vi "Generate Specific Result.vi"(8 "error in (no error)":errorcluster, 10 "Test Method":T4) -> (0 "error out":errorcluster, 3 "Data":T1[](array[typedef])=[{"Name"="Test Case.lvclass:Test Failing Test.vi", "Description"="Description", "Status"=enum."Failed", "Result Type"=enum."Fail", "Execution Time"=0.0, "Data"={"Expected"=variant, "Actual"=variant, "Delta"=variant}}, {"Name"="Test Case.lvclass:Test Failing Test.vi", "Description"="Failed:\nDescription\nMessage", "Status"=enum."Failed", "Result Type"=enum."Test Case", "Execution Time"=0.013, "Data"={"Expected"=variant, "Actual"=variant, "Delta"=variant}}, {"Name"="Test Case.lvclass:Test Passing Test.vi", "Description"="Description", "Status"=enum."Passed", "Result Type"=enum."Pass", "Execution Time"=0.0, "Data"={"Expected"=variant, "Actual"=variant, "Delta"=variant}}, {"Name"="Test Case.lvclass:Test Passing Test.vi", "Description"="Passed:\nDescription\nMessage", "Status"=enum."Passed", "Result Type"=enum."Test Case", "Execution Time"=0.022, "Data"={"Expected"=variant, "Actual"=variant, "Delta"=variant}}, {"Name"="Test Case.lvclass", "Description"="", "Status"=enum."Failed", "Result Type"=enum."Test Suite", "Execution Time"=0.0, "Data"={"Expected"=variant, "Actual"=variant, "Delta"=variant}}, {"Name"="Test Suite", "Description"="", "Status"=enum."Failed", "Result Type"=enum."Test Suite", "Execution Time"=0.0, "Data"={"Expected"=variant, "Actual"=variant, "Delta"=variant}}])   [LabVIEW 2020, in "Text Report Test.lvclass"]
uses:
  Text Report Test.lvclass
  source/Core/Result/Result.ctl
  source/Core/Result/Status.ctl
  source/Core/Result/Type.ctl
  Test Doubles/Test Case Test Double/Methods.ctl
  Test Doubles/Test Case Test Double/Test Case Test Double.lvclass
  source/Core/Result/Result.lvlib
  source/LUnit Test Case.lvclass
panel:
  out "Results":cluster{"Results":T1[]}[](array[cluster])
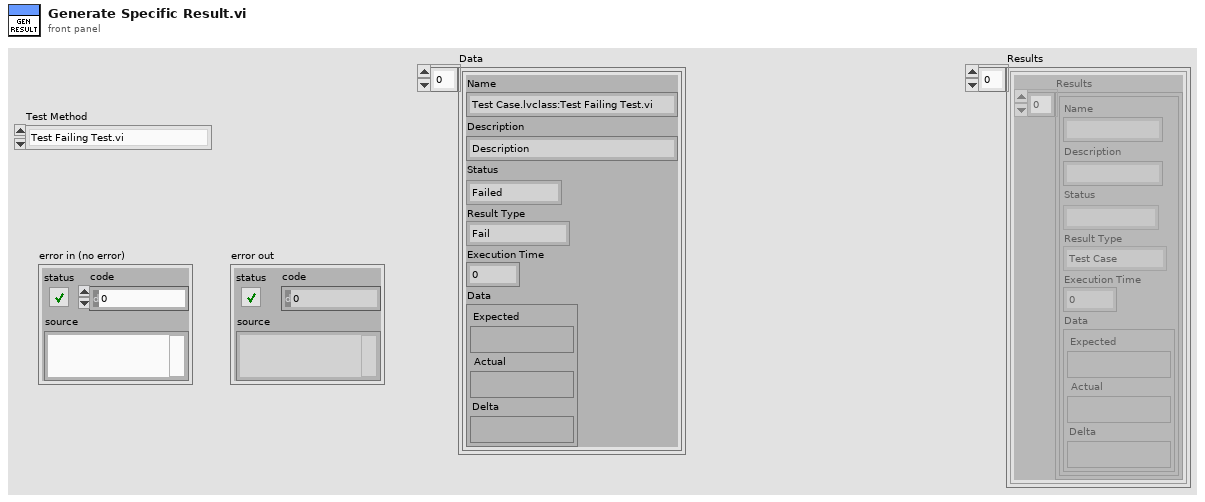
[diagram p1: front panel]
types:
  T1 = typedef "Result.lvlib/Result.ctl" = cluster{"Name":string, "Description":string, "Status":T2, "Result Type":T3, "Execution Time":dbl, "Data":cluster{"Expected":variant, "Actual":variant, "Delta":variant}}
  T2 = typedef "Result.lvlib/Status.ctl" = enum16{"", "Passed", "Failed", "Error", "Skipped", "Setup Error", "Broken", "Teardown Error"}
  T3 = typedef "Result.lvlib/Type.ctl" = enum16{"Test Case", "Test Suite", "Test Run", "Pass", "Fail", "Skip", "Pass if", "Fail if", "Pass if Error", "Fail if Error", "Pass if Equal", "Fail if Equal"}
  T4 = typedef "Test Case Test Double.lvclass/Methods.ctl" = enum16{"Test Failing Test.vi", "Test Passing Test.vi", "Test Error Test.vi", "Test Skip Test.vi", "Test Passing Pass If Test.vi", "Test Failing Pass If Test.vi", "Test Failing Fail If Test.vi", "Test Passing Fail If Test.vi", "Test Passing Pass If Error Test.vi", "Test Failing Pass If Error Test.vi", "Test Passing Fail If Error Test.vi", "Test Failing Fail If Error Test.vi", "Test Passing Pass If Equal Test.vi", "Test Failing Pass If Equal Test.vi", "Test Failing Fail If Equal Test.vi", "Test Passing Fail If Equal Test.vi", "Freezing Test.vi", "Test Pass on Expected Error Code.vi", "Test Error on Unexpected Error Code.vi", "Test Fail on Expected Error Code.vi", "Test Error when Fail on Unexpected Error Code.vi", "Test Pass on Expected Element in Array.vi", "Test Fail on Expected Element Not in Array.vi", "Test Pass on Expected Element in Set.vi", "Test Fail on Expected Element Not in Set.vi", "Test Pass on Expected Element in Map.vi", "Test Fail on Expected Element Not in Map.vi", "Test Fail on Unexpected Element in Array.vi", "Test Pass on Unexpected Element Not in Array.vi", "Test Fail if Unexpected Element in Set.vi", "Test Pass if Unexpected Element Not in Set.vi", "Test Fail if Unexpected Element in Map.vi", "Test Pass if Unexpected Element Not in Map.vi", "Test Pass on Expected Element in Array of Clusters.vi", "Test Pass on Expected Element Not in Array of Clusters.vi", "Test Matching String Test.vi", "Test Not Matching String Test.vi", "Verify Passing.vi", "Without Prefix.vi", "Private VI.vi"}
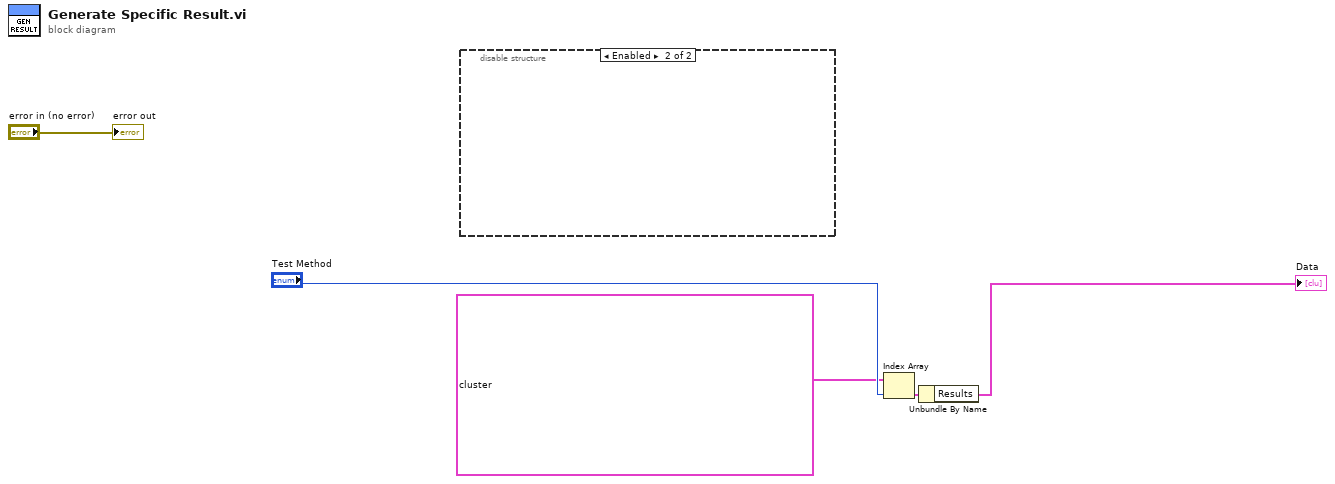
[diagram p0: block diagram]
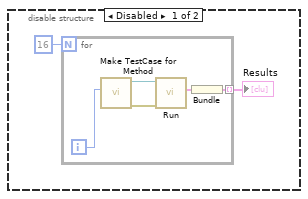
[diagram p2: hidden frame]
diagram:
  n1 = disable-structure shown="Enabled" {
    frame Disabled {
      n2 = for {
        N: 16 -> [_]
        tunnel: [w9] -> w6 mode=indexing
        i -> [w10]
        n3 = call "Make TestCase for Method.vi"("Test Method"=w10) -> ("error out"=w11:errorcluster, "LUnit Test Case V2 out"=w12:refnum<class "LUnit Test Case.lvclass">)  [unwired: 9 in]
        n4 = call-dynamic "Run.vi"("error in (no error)"=w11, "LUnit Test Case In"=w12) -> ("Results"=w8:T1[])  [unwired: 6 in, 3 out]
        n5 = Bundle("Results"=w8) -> (w9:cluster{"Results":T1[]})  [unwired: 1 in]
      }
      "Results" <- w6
    }
    frame Enabled {
    }
  }
  n6 = Index Array(array=cluster{"Results":T1[]}[] [{"Results"=[{"Name"="Test Case Test Double.lvclass:Test Failing Test.vi", "Description"="Description", "Status"=enum."Failed", "Result Type"=enum."Fail", "Execution Time"=0.0, "Data"={"Expected"=variant, "Actual"=variant, "Delta"=variant}}, {"Name"="Test Case Test Double.lvclass:Test Failing Test.vi", "Description"="Failed:\nMessage", "Status"=enum."Failed", "Result Type"=enum."Test Case", "Execution Time"=0.067, "Data"={"Expected"=variant, "Actual"=variant, "Delta"=variant}}]}, {"Results"=[{"Name"="Test Case Test Double.lvclass:Test Passing Test.vi", "Description"="", "Status"=enum."Passed", "Result Type"=enum."Pass", "Execution Time"=0.0, "Data"={"Expected"=variant, "Actual"=variant, "Delta"=variant}}, {"Name"="Test Case Test Double.lvclass:Test Passing Test.vi", "Description"="Passed", "Status"=enum."Passed", "Result Type"=enum."Test Case", "Execution Time"=0.051, "Data"={"Expected"=variant, "Actual"=variant, "Delta"=variant}}]}, {"Results"=[{"Name"="Test Case Test Double.lvclass:Test Error Test.vi", "Description"="Source", "Status"=enum."Error", "Result Type"=enum."Test Case", "Execution Time"=0.0, "Data"={"Expected"=variant, "Actual"=variant, "Delta"=variant}}]}, {"Results"=[{"Name"="Test Case Test Double.lvclass:Test Skip Test.vi", "Description"="Description", "Status"=enum."Skipped", "Result Type"=enum."Skip", "Execution Time"=0.0, "Data"={"Expected"=variant, "Actual"=variant, "Delta"=variant}}, {"Name"="Test Case Test Double.lvclass:Test Skip Test.vi", "Description"="Skipped:\nDescription\nMessage", "Status"=enum."Skipped", "Result Type"=enum."Test Case", "Execution Time"=0.07, "Data"={"Expected"=variant, "Actual"=variant, "Delta"=variant}}]}, {"Results"=[{"Name"="Test Case Test Double.lvclass:Test Passing Pass If Test.vi", "Description"="Description", "Status"=enum."Passed", "Result Type"=enum."Pass if", "Execution Time"=0.0, "Data"={"Expected"=variant, "Actual"=variant, "Delta"=variant}}, {"Name"="Test Case Test Double.lvclass:Test Passing Pass If Test.vi", "Description"="Passed:\nDescription\nMessage", "Status"=enum."Passed", "Result Type"=enum."Test Case", "Execution Time"=0.048, "Data"={"Expected"=variant, "Actual"=variant, "Delta"=variant}}]}, {"Results"=[{"Name"="Test Case Test Double.lvclass:Test Failing Pass If Test.vi", "Description"="Description", "Status"=enum."Failed", "Result Type"=enum."Pass if", "Execution Time"=0.0, "Data"={"Expected"=variant, "Actual"=variant, "Delta"=variant}}, {"Name"="Test Case Test Double.lvclass:Test Failing Pass If Test.vi", "Description"="Failed:\nDescription\nMessage", "Status"=enum."Failed", "Result Type"=enum."Test Case", "Execution Time"=0.042, "Data"={"Expected"=variant, "Actual"=variant, "Delta"=variant}}]}, {"Results"=[{"Name"="Test Case Test Double.lvclass:Test Failing Fail If Test.vi", "Description"="Description", "Status"=enum."Failed", "Result Type"=enum."Fail if", "Execution Time"=0.0, "Data"={"Expected"=variant, "Actual"=variant, "Delta"=variant}}, {"Name"="Test Case Test Double.lvclass:Test Failing Fail If Test.vi", "Description"="Failed:\nDescription\nMessage", "Status"=enum."Failed", "Result Type"=enum."Test Case", "Execution Time"=0.05, "Data"={"Expected"=variant, "Actual"=variant, "Delta"=variant}}]}, {"Results"=[{"Name"="Test Case Test Double.lvclass:Test Passing Fail If Test.vi", "Description"="Description", "Status"=enum."Passed", "Result Type"=enum."Fail if", "Execution Time"=0.0, "Data"={"Expected"=variant, "Actual"=variant, "Delta"=variant}}, {"Name"="Test Case Test Double.lvclass:Test Passing Fail If Test.vi", "Description"="Passed:\nDescription\nMessage", "Status"=enum."Passed", "Result Type"=enum."Test Case", "Execution Time"=0.052, "Data"={"Expected"=variant, "Actual"=variant, "Delta"=variant}}]}, {"Results"=[{"Name"="Test Case Test Double.lvclass:Test Passing Pass If Error Test.vi", "Description"="Description", "Status"=enum."Passed", "Result Type"=enum."Pass if Error", "Execution Time"=0.0, "Data"={"Expected"=variant, "Actual"=variant, "Delta"=variant}}, {"Name"="Test Case Test Double.lvclass:Test Passing Pass If Error Test.vi", "Description"="Passed:\nDescription\nError 42 occured: \"Error\"", "Status"=enum."Passed", "Result Type"=enum."Test Case", "Execution Time"=0.037, "Data"={"Expected"=variant, "Actual"=variant, "Delta"=variant}}]}, {"Results"=[{"Name"="Test Case Test Double.lvclass:Test Failing Pass If Error Test.vi", "Description"="Description", "Status"=enum."Failed", "Result Type"=enum."Pass if Error", "Execution Time"=0.0, "Data"={"Expected"=variant, "Actual"=variant, "Delta"=variant}}, {"Name"="Test Case Test Double.lvclass:Test Failing Pass If Error Test.vi", "Description"="Failed:\nDescription\nNo error occured.", "Status"=enum."Failed", "Result Type"=enum."Test Case", "Execution Time"=0.043, "Data"={"Expected"=variant, "Actual"=variant, "Delta"=variant}}]}, {"Results"=[{"Name"="Test Case Test Double.lvclass:Test Passing Fail If Error Test.vi", "Description"="Description", "Status"=enum."Passed", "Result Type"=enum."Fail if Error", "Execution Time"=0.0, "Data"={"Expected"=variant, "Actual"=variant, "Delta"=variant}}, {"Name"="Test Case Test Double.lvclass:Test Passing Fail If Error Test.vi", "Description"="Passed:\nDescription\nNo error occured.", "Status"=enum."Passed", "Result Type"=enum."Test Case", "Execution Time"=0.042, "Data"={"Expected"=variant, "Actual"=variant, "Delta"=variant}}]}, {"Results"=[{"Name"="Test Case Test Double.lvclass:Test Failing Fail If Error Test.vi", "Description"="Description", "Status"=enum."Failed", "Result Type"=enum."Fail if Error", "Execution Time"=0.0, "Data"={"Expected"=variant, "Actual"=variant, "Delta"=variant}}, {"Name"="Test Case Test Double.lvclass:Test Failing Fail If Error Test.vi", "Description"="Failed:\nDescription\nError 42 occured: \"Error\"", "Status"=enum."Failed", "Result Type"=enum."Test Case", "Execution Time"=0.036, "Data"={"Expected"=variant, "Actual"=variant, "Delta"=variant}}]}, {"Results"=[{"Name"="Test Case Test Double.lvclass:Test Passing Pass If Equal Test.vi", "Description"="Description", "Status"=enum."Passed", "Result Type"=enum."Pass if Equal", "Execution Time"=0.0, "Data"={"Expected"=variant, "Actual"=variant, "Delta"=variant}}, {"Name"="Test Case Test Double.lvclass:Test Passing Pass If Equal Test.vi", "Description"="Passed:\nDescription\nExpected: Equal\nActual:   Equal", "Status"=enum."Passed", "Result Type"=enum."Test Case", "Execution Time"=0.056, "Data"={"Expected"=variant, "Actual"=variant, "Delta"=variant}}]}, {"Results"=[{"Name"="Test Case Test Double.lvclass:Test Failing Pass If Equal Test.vi", "Description"="Description", "Status"=enum."Failed", "Result Type"=enum."Pass if Equal", "Execution Time"=0.0, "Data"={"Expected"=variant, "Actual"=variant, "Delta"=variant}}, {"Name"="Test Case Test Double.lvclass:Test Failing Pass If Equal Test.vi", "Description"="Failed:\nDescription\nExpected: Equal\nActual:   Not Equal", "Status"=enum."Failed", "Result Type"=enum."Test Case", "Execution Time"=0.045, "Data"={"Expected"=variant, "Actual"=variant, "Delta"=variant}}]}, {"Results"=[{"Name"="Test Case Test Double.lvclass:Test Failing Fail If Equal Test.vi", "Description"="Description", "Status"=enum."Failed", "Result Type"=enum."Fail if Equal", "Execution Time"=0.0, "Data"={"Expected"=variant, "Actual"=variant, "Delta"=variant}}, {"Name"="Test Case Test Double.lvclass:Test Failing Fail If Equal Test.vi", "Description"="Failed:\nDescription\nExpected: Equal\nActual:   Equal", "Status"=enum."Failed", "Result Type"=enum."Test Case", "Execution Time"=0.046, "Data"={"Expected"=variant, "Actual"=variant, "Delta"=variant}}]}, {"Results"=[{"Name"="Test Case Test Double.lvclass:Test Passing Fail If Equal Test.vi", "Description"="Description", "Status"=enum."Passed", "Result Type"=enum."Fail if Equal", "Execution Time"=0.0, "Data"={"Expected"=variant, "Actual"=variant, "Delta"=variant}}, {"Name"="Test Case Test Double.lvclass:Test Passing Fail If Equal Test.vi", "Description"="Passed:\nDescription\nExpected: Equal\nActual:   Not Equal", "Status"=enum."Passed", "Result Type"=enum."Test Case", "Execution Time"=0.04, "Data"={"Expected"=variant, "Actual"=variant, "Delta"=variant}}]}] ("Results"), index="Test Method") -> (element=w4:cluster{"Results":T1[]})
  n7 = Unbundle By Name(w4) -> ("Results"=→"Data":T1[])
  "error out" <- "error in (no error)"
